vi "Fixup tagValue Decode Error.vi"(6 "tagValue":T1={"type"="tagValue", "tag"="", "value"="", "t"=""}, 8 "error in (no error)":errorcluster) -> (0 "error out":errorcluster)   [LabVIEW 2017]
uses:
  Common/Typedefs/tagValue.ctl
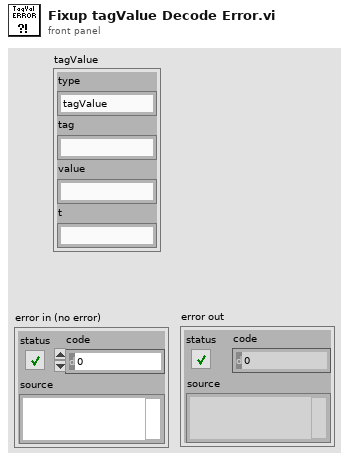
[diagram p1: front panel]
types:
  T1 = typedef "tagValue.ctl" = cluster{"type":string, "tag":string, "value":string, "t":string}
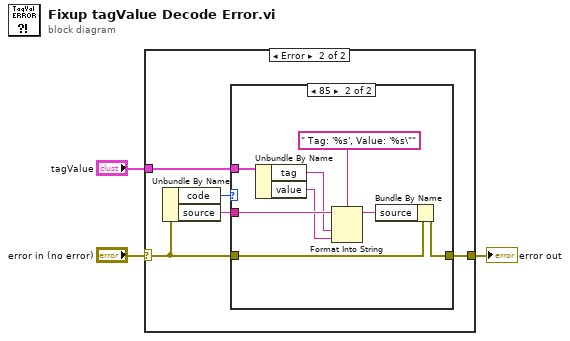
[diagram p0: block diagram]
diagram:
  n1 = case shown="Error" "error in (no error)" {
    selector: "error in (no error)" -> [w4 w8]
    tunnel: [w4 w7] -> w2
    tunnel: "tagValue" -> [_ w5]
    frame No Error {
    }
    frame Error {
      n2 = Unbundle By Name(w8) -> ("code"=w9:i32, "source"=w6:string)
      n3 = case shown="85" w9 {
        tunnel: w8 -> [w10 w18]
        tunnel: [w10 w17] -> w7
        tunnel: w6 -> [_ w16]
        tunnel: w5 -> [_ w13]
        frame Default {
        }
        frame 85 {
          n4 = Unbundle By Name(w13) -> ("tag"=w12:string, "value"=w11:string)
          n5 = Format Into String(format string=" Tag: '%s', Value: '%s\"", initial string=w16, w12, w11) -> (resulting string=w15:string)  [unwired: 1 in, 1 out]
          n6 = Bundle By Name(cluster=w18, "source"=w15) -> (w17:errorcluster)
        }
      }
    }
  }
  "error out" <- w2
